vi "Send.vi"(8 "Is Priority":bool, 9 "Msg":refnum<class "Msg.lvclass">, 10 "Msg Event":refnum<user-event>) -> (0 "error out":errorcluster)   [LabVIEW 2021, in "jettl.lvlib" / "Temporary Actor.lvlib" / "jettl Actor.lvclass"]
uses:
  jettl Actor.lvclass
  Msg/Msg.lvclass
  <vilib>/event_ctls.llb/usereventprio.ctl
  jettl Actor.lvclass/jettl Actor.ctl
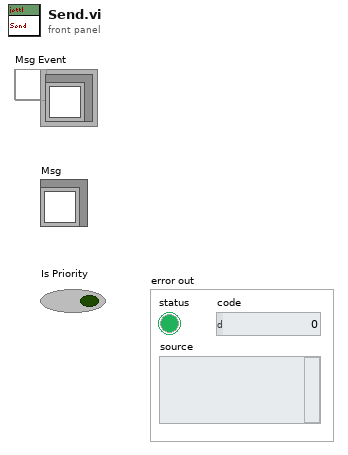
[diagram p1: front panel]
types:
  T1 = typedef "usereventprio.ctl" = enum32{"high priority", "normal priority"}
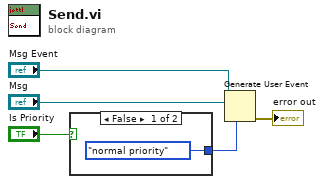
[diagram p0: block diagram]
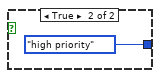
[diagram p2: hidden frame]
diagram:
  n1 = case shown="False" "Is Priority" {
    tunnel: [usereventprio."normal priority" ("priority (normal)") usereventprio."high priority" ("priority (normal)")] -> w5
    frame False {
    }
    frame True {
    }
  }
  n2 = Generate User Event(priority (normal)=w5, user event="Msg Event", event data cluster="Msg") -> (error out=→"error out":errorcluster)  [unwired: 1 in, 1 out]
